vi "Scope Instrument UI.vi"() -> ()   [LabVIEW 2025, in "Scope.lvlib" / "Scope Instrument.lvclass"]
doc: "Copyright 2017 National Instruments Corporation\n\nLicensed under the Apache License, Version 2.0 (the \"License\"); you may not use this file except in compliance with the License. You may obtain a copy of the License at http://www.apache.org/licenses/LICENSE-2.0\nUnless required by applicable law or agreed to in writing, software distributed under the License is distributed on an \"AS IS\" BASIS, WITHOUT WARRANTIES OR CONDITIONS OF ANY KIND, either express or implied. See the License for the specific language governing permissions and limitations under the License."
uses:
  Scope Instrument.lvclass
  Users/Public/Documents/Sandia National Labs/TSS Plugin/CEF.lvlibp/Node/NodeRef.ctl
  Users/Public/Documents/Sandia National Labs/TSS Plugin/CEF.lvlibp/Node/CEF_Node.lvclass
  Users/Public/Documents/Sandia National Labs/TSS Plugin/CEF.lvlibp/Node/mainQref.ctl
  Users/Public/Documents/Sandia National Labs/TSS Plugin/CEF.lvlibp/Node/UserEventRef.ctl
  Users/Public/Documents/Sandia National Labs/TSS Plugin/Abstract Engine.lvlibp/Instrument configuration/Default Instrument.ctl
  Scope configuration/Scope Instrument Setting.ctl
  C:/Users/Public/Documents/Sandia National Labs/TSS Plugin/CEF.lvlibp/Node/CEF_Node.lvclass
  Scope Instrument.lvclass/Scope Instrument.ctl
  Scope configuration/Scope configuration.lvclass/Scope configuration.ctl
  Scope configuration/Read Scope Setting.vi
  Scope configuration/Write Scope Setting.vi
  <vilib>/Utility/error.llb/Trim Whitespace One-Sided.vi
  Scope configuration/Scope configuration.lvclass
  C:/Users/Public/Documents/Sandia National Labs/TSS Plugin/Abstract Engine.lvlibp/Instrument configuration/Instrument configuration.lvclass
  Users/Public/Documents/Sandia National Labs/TSS Plugin/Abstract Engine.lvlibp/Instrument configuration/Read Instrument Setting.vi
  Users/Public/Documents/Sandia National Labs/TSS Plugin/Abstract Engine.lvlibp/Instrument configuration/Write Instrument Setting.vi
  Users/Public/Documents/Sandia National Labs/TSS Plugin/Abstract Engine.lvlibp/Instrument configuration/Instrument configuration.lvclass
panel:
  in  "Scope":cluster{"Default":T1, "Setting":T2}={"Default"={"Type"="Foundation Bus", "Address"="None", "SW Alias"="None", "Description"="* Type = Class", "Enabled"=TRUE}, "Setting"={"Sampling Rate"=10000000.0, "Number of Samples"=1000000, "Type"="Window - Entering", "Pretrigger"=50.0, "Source"="CH0", "Level 1"=1.0, "Level 2"=0.0, "Trigger Coupling"="DC", "TrigDest"="None", "Group"="None"}} {"Setting"."Level 2" format="%#_6p"; "Setting"."Level 1" format="%#_6p"; "Setting"."Pretrigger" format="%#_f"; "Setting"."Number of Samples" format="%#_6p"; "Setting"."Sampling Rate" format="%#_6p"}
  in  "user event":T3
  in  "main queue":T4
  in  "node ref":T5
  # "Trigger"
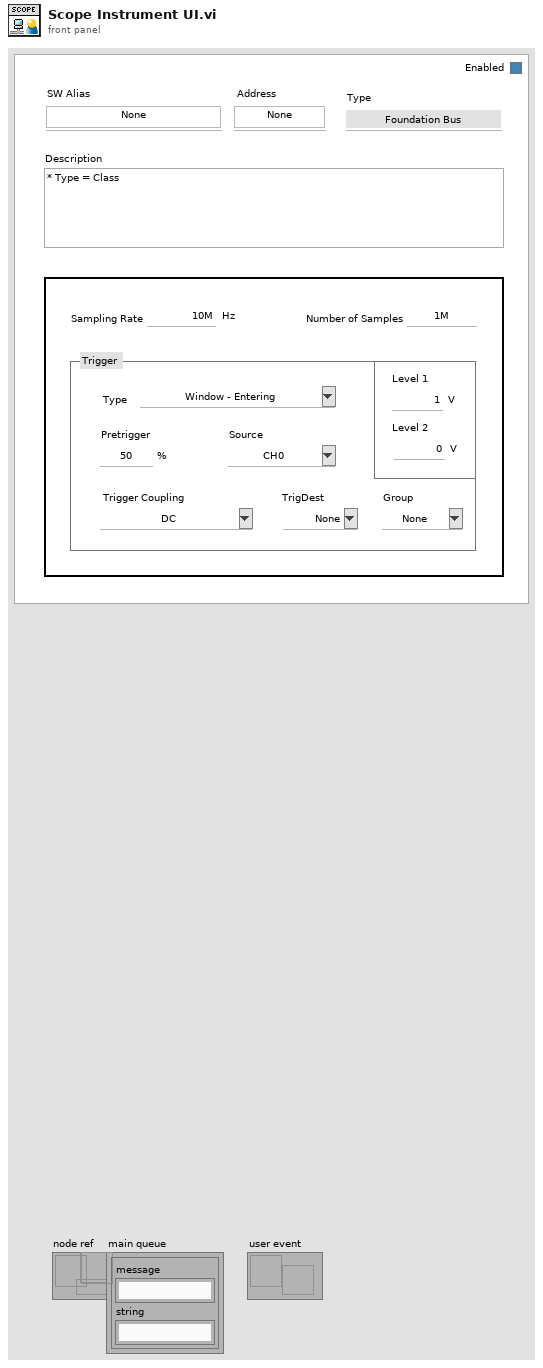
[diagram p1: front panel]
types:
  T1 = typedef "Abstract Engine.lvlibp/Instrument configuration.lvclass/Default Instrument.ctl" = cluster{"Type":string, "Address":string, "SW Alias":string, "Description":string, "Enabled":bool}
  T2 = typedef "Scope.lvlib/Scope configuration.lvclass/Scope Instrument Setting.ctl" = cluster{"Sampling Rate":dbl, "Number of Samples":u32, "Type":string, "Pretrigger":dbl, "Source":string, "Level 1":dbl, "Level 2":dbl, "Trigger Coupling":string, "TrigDest":string, "Group":string}
  T3 = typedef "CEF.lvlibp/CEF_Node.lvclass/UserEventRef.ctl" = refnum<user-event>
  T4 = typedef "CEF.lvlibp/CEF_Node.lvclass/mainQref.ctl" = refnum<queue>
  T5 = typedef "CEF.lvlibp/CEF_Node.lvclass/NodeRef.ctl" = refnum<data-value>
  T6 = cluster{"Instrument Setting":T1, "Scope Setting":T2}
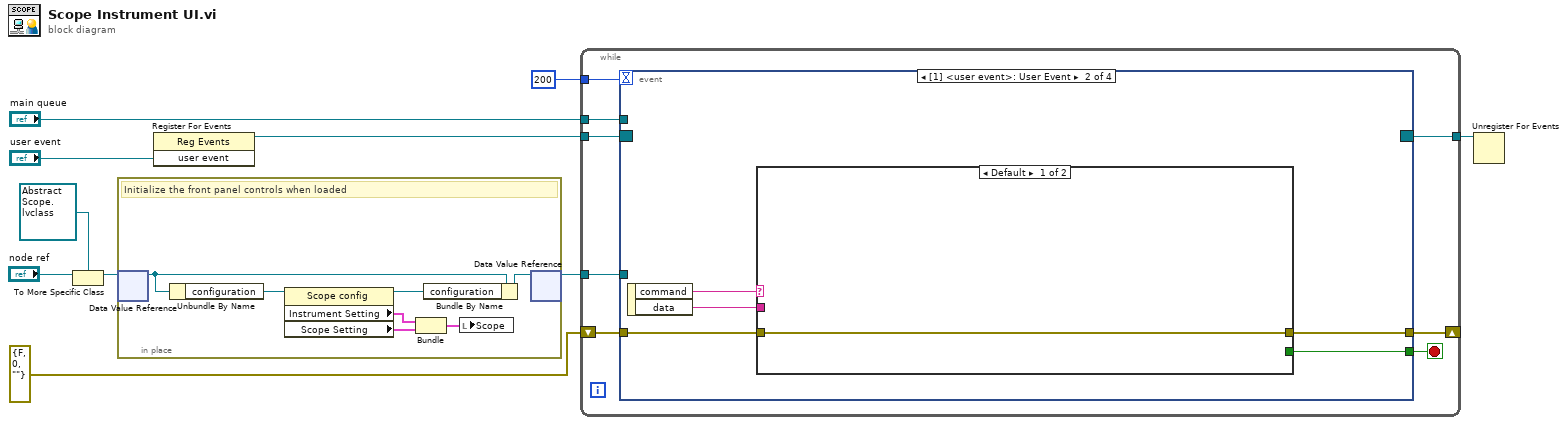
[diagram p0: block diagram]
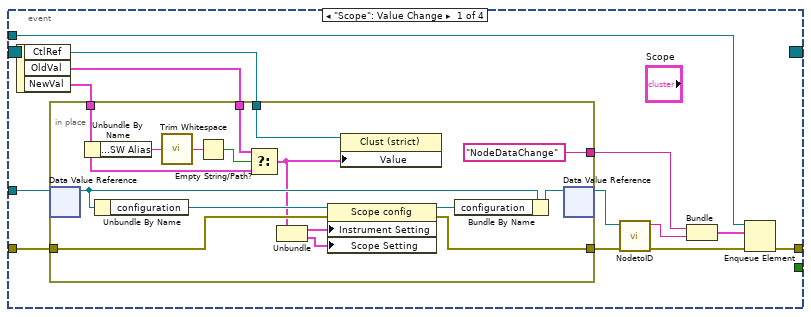
[diagram p2: hidden frame]
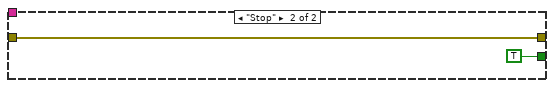
[diagram p3: hidden frame]
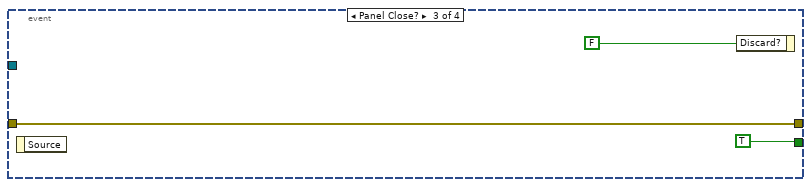
[diagram p4: hidden frame]
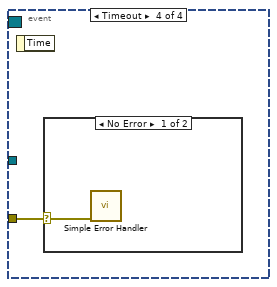
[diagram p5: hidden frame]
diagram:
  n1 = To More Specific Class(target class=refnum<data-value> refnum ("data value reference"), reference="node ref") -> (specific class reference=w6:refnum<data-value>)  [unwired: 1 in, 1 out]
  n2 = in-place {
    # "Initialize the front panel controls when loaded"
    n3 = in-place-dvr #1(w6) -> (w17:refnum<class "Scope Instrument.lvclass">)  [unwired: 1 out]
    n4 = Unbundle By Name(w17) -> ("configuration"=w16:refnum<class "Scope configuration.lvclass">)
    n5 = property class="Scope config"(reference=w16) -> (reference out=w14:refnum<class "Scope configuration.lvclass">, "Instrument Setting"=w11:T1, "Scope Setting"=w13:T2)  [unwired: 1 in, 1 out]
    n6 = Bundle("Instrument Setting"=w11, "Scope Setting"=w13) -> (w12:T6)  [unwired: 1 in]
    n7 = Bundle By Name(cluster=w17, "configuration"=w14) -> (w15:refnum<class "Scope Instrument.lvclass">)
    n8 = local write "Scope"(w12) -> ()
    n9 = in-place-dvr #1(w15) -> (w5:refnum<data-value>)  [unwired: 1 out]
  }
  n10 = register-events("user event") -> (reference out=w8:refnum<event-registration>)  [unwired: 2 in, 1 out]
  n11 = while {
    tunnel: "main queue" -> [w24]
    tunnel: w5 -> [w23]
    tunnel: w8 -> [w21]
    tunnel: [w20] -> w7
    tunnel: 200 -> [w18]
    shift-right: [w22] -> _
    shift-left: errorcluster {"status"=FALSE, "code"=0, "source"=""} ("error out") -> [w25]
    stop <- w19 stop-if-true
    n12 = event shown="[1] <user event>: User Event" {
      selector: w21 -> [_ _ _ _]
      dyn-events: [_ _ _ _] -> w20
      timeout: w18 -> [_ _ _ _]
      tunnel: [w38 w56 w63 _] -> w22
      tunnel: w25 -> [w35 w57 w63 w66]
      tunnel: w24 -> [w37 _ _ _]
      tunnel: w23 -> [w36 _ _ _]
      tunnel: [_ w55 TRUE _] -> w19
      event "Scope": Value Change {
        n13 = event-data() -> ("CtlRef"=w31:refnum<vi>, "OldVal"=w32:cluster{"Default":T1, "Setting":T2}, "NewVal"=w33:cluster{"Default":T1, "Setting":T2})  [unwired: 1 in]
        n14 = in-place {
          in-place-border: w35 -> [w53]
          in-place-border: [w50] -> w27
          in-place-border: w33 -> [w40]
          in-place-border: w32 -> [w49]
          in-place-border: w31 -> [w48]
          in-place-border: ["NodeDataChange" ("Message Name")] -> w30
          n15 = in-place-dvr #2(w36) -> (w54:refnum<class "Scope Instrument.lvclass">)  [unwired: 1 out]
          n16 = Unbundle By Name(w40) -> ("Default.SW Alias"=w41:string)
          n17 = Unbundle By Name(w54) -> ("configuration"=w47:refnum<class "Scope configuration.lvclass">)
          n18 = call <vilib>:"Trim Whitespace.vi"("string"=w41) -> ("trimmed string"=w42:string)  [unwired: 1 in]
          n19 = Empty String/Path?(string/path=w42) -> (empty?=w39:bool)
          n20 = Select(t=w49, s=w39, f=w40) -> (s? t:f=w46:cluster{"Default":T1, "Setting":T2})
          n21 = Unbundle(w46) -> ("Default"=w45:T1, "Setting"=w44:T2)
          n22 = property class="Scope config"(reference=w47, error in=w53, "Instrument Setting"=w45, "Scope Setting"=w44) -> (reference out=w51:refnum<class "Scope configuration.lvclass">, error out=w50:errorcluster)
          n23 = property class="Clust (strict)"(reference=w48, "Value"=w46) -> ()  [unwired: 1 in, 2 out]
          n24 = Bundle By Name(cluster=w54, "configuration"=w51) -> (w52:refnum<class "Scope Instrument.lvclass">)
          n25 = in-place-dvr #2(w52) -> (w34:refnum<data-value>)  [unwired: 1 out]
        }
        n26 = call "NodetoID.vi"("error in"=w27, "node ref"=w34) -> ("error out"=w26:errorcluster, "ID"=w29:string)  [unwired: 8 in]
        n27 = Bundle("Message Name"=w30, "ID"=w29) -> (w28:cluster{"Message Name":string, "ID":string})  [unwired: 1 in]
        n28 = Enqueue Element(queue=w37, element=w28, error in (no error)=w26) -> (error out=w38:errorcluster)  [unwired: 1 in, 2 out]
      }
      event User Event {
        n29 = event-data() -> ("command"=w59:string, "data"=w58:string)  [unwired: 1 in]
        n30 = case shown="Default" w59 {
          tunnel: w58 -> [_ _]
          tunnel: w57 -> [w60 w61]
          tunnel: [w60 w61] -> w56
          tunnel: [_ TRUE] -> w55
          frame Default {
          }
          frame "Stop" {
          }
        }
      }
      event Panel Close? {
        n31 = event-data() -> ()  [unwired: 1 in, 1 out]
        n32 = event-data("Discard?"=FALSE) -> ()  [unwired: 1 in, 1 out]
      }
      event Timeout {
        n33 = event-data() -> ()  [unwired: 1 in, 1 out]
        n34 = case shown="No Error" w66 {
          selector: w66 -> [w67 _]
          frame No Error {
            n35 = call <vilib>:"Simple Error Handler.vi"("error in (no error)"=w67) -> ()  [unwired: 4 in, 5 out]
          }
          frame Error {
          }
        }
      }
    }
  }
  n36 = Unregister For Events(event registration refnum=w7) -> ()  [unwired: 1 in, 1 out]
